vi "Log from event queue.vi"() -> ()   [LabVIEW 2020]
uses:
  Event log.ctl
  Global Variables/General Globals.vi
panel:
  out "Numeric":i32
  out "x-y":dbl
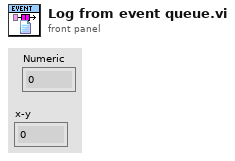
[diagram p1: front panel]
types:
  T1 = enum16{"Create/Open File", "Write File", "Close file"}
  T2 = typedef "Event log.ctl" = cluster{"Time":timestamp, "Event":string[]}
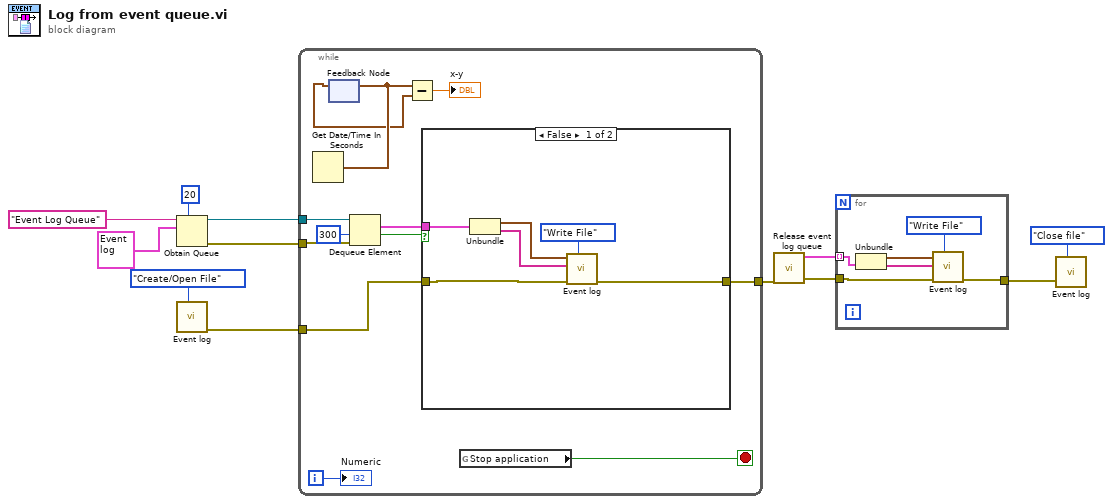
[diagram p0: block diagram]
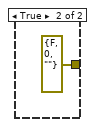
[diagram p2: hidden frame]
diagram:
  n1 = Obtain Queue(max queue size (-1, unlimited)=20, name (unnamed)="Event Log Queue", element data type=T2 {"Time"=timestamp(0 s since 1904-01-01), "Event"=[]}) -> (queue out=w8:refnum<queue>, error out=w9:errorcluster)  [unwired: 2 in, 1 out]
  n2 = call "Event log.vi"("File Ops"=T1."Create/Open File") -> ("error out 2"=w6:errorcluster)  [unwired: 10 in]
  n3 = while {
    tunnel: w9 -> [w24]
    tunnel: w8 -> [w23]
    tunnel: w6 -> [w13]
    tunnel: [w18] -> w5
    i -> [w17]
    stop <- w20 stop-if-true
    n4 = Get Date/Time In Seconds() -> (seconds since 1Jan1904=w16:timestamp)
    n5 = feedback-in #1(w16) -> ()
    n6 = feedback #1() -> (w15:timestamp)  [unwired: 1 in]
    n7 = Dequeue Element(queue=w23, timeout in ms (-1)=300, error in (no error)=w24) -> (element=w19:T2, timed out?=w21:bool)  [unwired: 2 out]
    n8 = Subtract(x=w16, y=w15) -> (x-y=→"x-y":dbl)
    n9 = case shown="False" w21 {
      tunnel: w19 -> [w29 _]
      tunnel: [w26 errorcluster {"status"=FALSE, "code"=0, "source"=""} ("error out 2")] -> w18
      tunnel: w13 -> [w25 _]
      frame False {
        n10 = Unbundle(w29) -> ("Time"=w28:timestamp, "Event"=w27:string[])
        n11 = call "Event log.vi"("File Ops"=T1."Write File", "error in (no error)"=w25, "Event Details"=w27, "time stamp"=w28) -> ("error out 2"=w26:errorcluster)  [unwired: 7 in]
      }
      frame True {
      }
    }
    n12 = global read "General Globals.vi" "Stop application"() -> (w20:bool)
    "Numeric" <- w17
  }
  n13 = call "Release event log queue.vi"("error in (no error)"=w5) -> ("error out"=w4:errorcluster, "remaining elements"=w1:T2[])  [unwired: 9 in]
  n14 = for {
    tunnel: w4 -> [w33]
    tunnel: [w32] -> w2
    tunnel: w1 -> [w34] mode=indexing
    n15 = Unbundle(w34) -> ("Time"=w36:timestamp, "Event"=w35:string[])
    n16 = call "Event log.vi"("File Ops"=T1."Write File", "error in (no error)"=w33, "Event Details"=w35, "time stamp"=w36) -> ("error out 2"=w32:errorcluster)  [unwired: 7 in]
  }
  n17 = call "Event log.vi"("File Ops"=T1."Close file", "error in (no error)"=w2) -> ()  [unwired: 9 in, 1 out]
